vi "CRYTS Step Unflatten.vi"(9 "Sequence Name":string, 10 "Version":u16, 11 "Flattened Steps":string) -> (3 "Unflattened Steps":T2[](array[typedef]) {"Repeat State Array"."Start" format="%#_5g"; "Y dB ref" format="%.1f"; "Y data" items=["dB", "Lin"]; "Start" format="%#_5g"})   [LabVIEW 2013]
uses:
  CRYSystem/Typedef Control/CRYStep.ctl
panel:
  in  "Version2,3":T1(array[cluster])
  in  "Version1":T3(array[cluster])
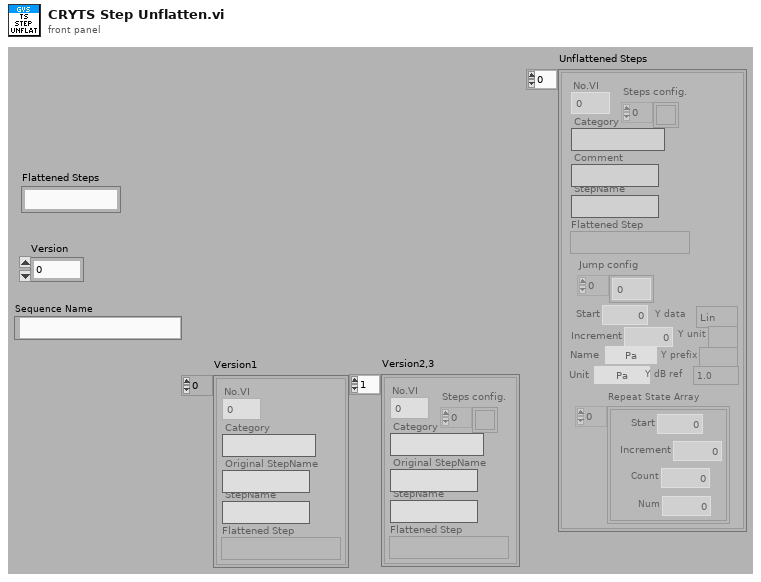
[diagram p1: front panel]
types:
  T1 = cluster{"No.VI":u16, "Category":string, "StepName":string, "Seq setup flattened":string, "Original StepName":string, "Steps config.":bool[]}[]
  T2 = typedef "CRYStep.ctl" = cluster{"No.VI":i32, "Category":string, "StepName":string, "Seq setup flattened":string, "Comment":string, "Steps config.":bool[], "Jump config":i32[], "Start":dbl, "Increment":dbl, "Name":string, "Unit":string, "Y data":u16, "Y prefix":string, "Y dB ref":dbl, "Y unit":string, "Repeat State Array":cluster{"Start":dbl, "Increment":dbl, "Count":i32, "Num":i32}[]}
  T3 = cluster{"No.VI":u16, "Category":string, "StepName":string, "Seq setup flattened":string, "Original StepName":string}[]
  T4 = cluster{"No.VI":i32, "Category":string, "StepName":string, "Seq setup flattened":string, "Original StepName":string, "Steps config.":bool[], "Jump config":i32[], "Start":dbl, "Increment":dbl, "Name":string, "Unit":string, "Y data":u16, "Y prefix":string, "Y dB ref":dbl, "Y unit":string}[]
  T5 = cluster{"Start":dbl, "Increment":dbl, "Count":i32, "Num":i32}[]
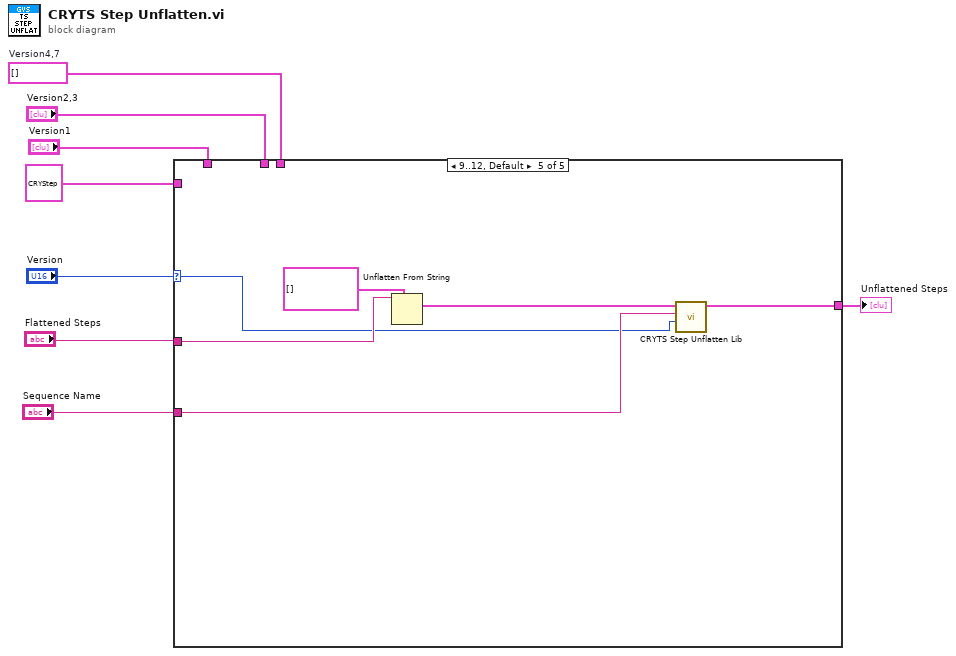
[diagram p0: block diagram]
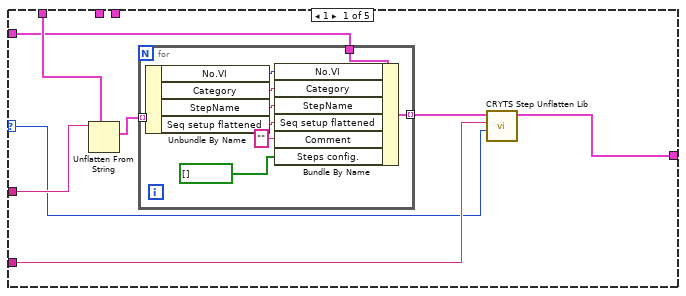
[diagram p2: hidden frame]
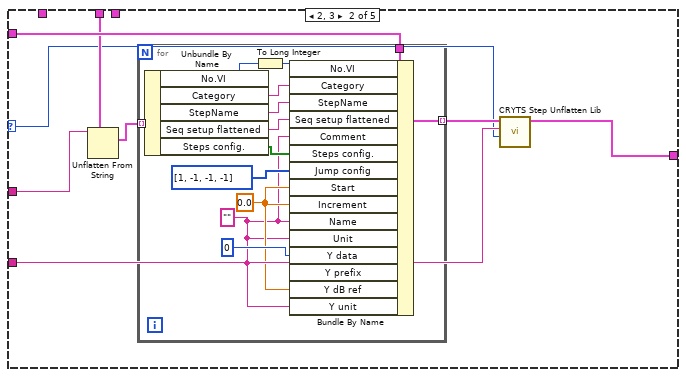
[diagram p3: hidden frame]
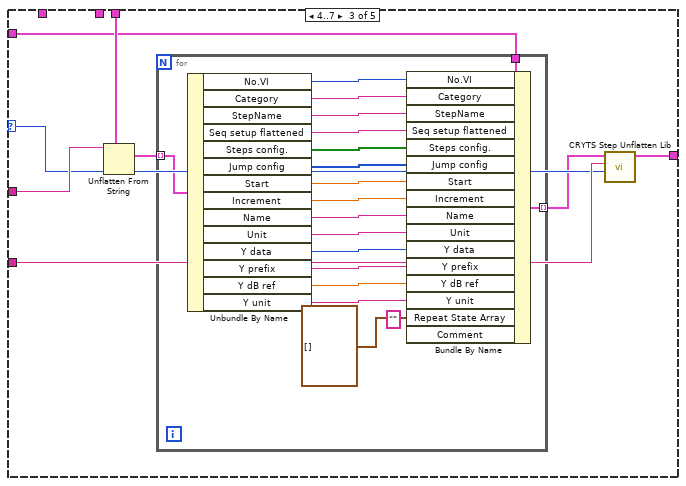
[diagram p4: hidden frame]
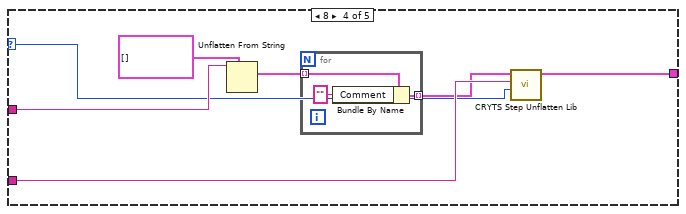
[diagram p5: hidden frame]
diagram:
  w1 = T4 []  # Version4,7
  n1 = case shown="9..12, Default" "Version" {
    selector: "Version" -> [w9 w26 w51 w76 w85]
    tunnel: [w11 w28 w53 w78 w87] -> w4
    tunnel: "Flattened Steps" -> [w16 w32 w54 w79 w88]
    tunnel: "Version1" -> [w14 _ _ _ _]
    tunnel: T2 {"No.VI"=0, "Category"="", "StepName"="", "Seq setup flattened"="", "Comment"="", "Steps config."=[], "Jump config"=[], "Start"=0.0, "Increment"=0.0, "Name"="", "Unit"="", "Y data"=0, "Y prefix"="", "Y dB ref"=0.0, "Y unit"="", "Repeat State Array"=[]} ("Step") -> [w13 w31 w48 _ _]
    tunnel: "Version2,3" -> [_ w30 _ _ _]
    tunnel: "Sequence Name" -> [w10 w27 w52 w77 w86]
    tunnel: w1 -> [_ _ w50 _ _]
    frame 1 {
      n2 = Unflatten From String(type=w14, binary string=w16) -> (value=w15:T3)  [unwired: 1 in, 4 out]
      n3 = for {
        tunnel: w15 -> [w24] mode=indexing
        tunnel: w13 -> [w25]
        tunnel: [w18] -> w12 mode=indexing
        n4 = Unbundle By Name(w24) -> ("No.VI"=w23:u16, "Category"=w22:string, "StepName"=w21:string, "Seq setup flattened"=w20:string)
        n5 = Bundle By Name(cluster=w25, "No.VI"=w23, "Category"=w22, "StepName"=w21, "Seq setup flattened"=w20, "Comment"="", "Steps config."=bool[] []) -> (w18:T2)
      }
      n6 = call "CRYTS Step Unflatten Lib.vi"("Version"=w9, "Sequence Name"=w10, "Steps In"=w12) -> ("Steps Out"=w11:T2[])  [unwired: 8 in]
    }
    frame 2, 3 {
      n7 = Unflatten From String(type=w30, binary string=w32) -> (value=w33:T1)  [unwired: 1 in, 4 out]
      n8 = for {
        tunnel: w33 -> [w45] mode=indexing
        tunnel: w31 -> [w46]
        tunnel: [w40] -> w29 mode=indexing
        w34 = "" ("Name")
        w36 = 0.0 ("Start")
        n9 = Unbundle By Name(w45) -> ("No.VI"=w44:u16, "Category"=w43:string, "StepName"=w42:string, "Seq setup flattened"=w41:string, "Steps config."=w39:bool[])
        n10 = To Long Integer(number=w44) -> (32bit integer=w35:i32)
        n11 = Bundle By Name(cluster=w46, "No.VI"=w35, "Category"=w43, "StepName"=w42, "Seq setup flattened"=w41, "Comment"=w34, "Steps config."=w39, "Jump config"=i32[] [1, -1, -1, -1], "Start"=w36, "Increment"=w36, "Name"=w34, "Unit"=w34, "Y data"=u16 0, "Y prefix"=w34, "Y dB ref"=w36, "Y unit"=w34) -> (w40:T2)
      }
      n12 = call "CRYTS Step Unflatten Lib.vi"("Version"=w26, "Sequence Name"=w27, "Steps In"=w29) -> ("Steps Out"=w28:T2[])  [unwired: 8 in]
    }
    frame 4..7 {
      n13 = Unflatten From String(type=w50, binary string=w54) -> (value=w49:T4)  [unwired: 1 in, 4 out]
      n14 = for {
        tunnel: w49 -> [w73] mode=indexing
        tunnel: w48 -> [w72]
        tunnel: [w71] -> w47 mode=indexing
        n15 = Unbundle By Name(w73) -> ("No.VI"=w70:i32, "Category"=w69:string, "StepName"=w68:string, "Seq setup flattened"=w67:string, "Steps config."=w66:bool[], "Jump config"=w65:i32[], "Start"=w64:dbl, "Increment"=w63:dbl, "Name"=w62:string, "Unit"=w61:string, "Y data"=w60:u16, "Y prefix"=w59:string, "Y dB ref"=w58:dbl, "Y unit"=w57:string)
        n16 = Bundle By Name(cluster=w72, "No.VI"=w70, "Category"=w69, "StepName"=w68, "Seq setup flattened"=w67, "Steps config."=w66, "Jump config"=w65, "Start"=w64, "Increment"=w63, "Name"=w62, "Unit"=w61, "Y data"=w60, "Y prefix"=w59, "Y dB ref"=w58, "Y unit"=w57, "Repeat State Array"=T5 [], "Comment"="") -> (w71:T2)
      }
      n17 = call "CRYTS Step Unflatten Lib.vi"("Version"=w51, "Sequence Name"=w52, "Steps In"=w47) -> ("Steps Out"=w53:T2[])  [unwired: 8 in]
    }
    frame 8 {
      n18 = Unflatten From String(type=T2[] [], binary string=w79) -> (value=w75:T2[])  [unwired: 1 in, 4 out]
      n19 = for {
        tunnel: w75 -> [w83] mode=indexing
        tunnel: [w81] -> w74 mode=indexing
        n20 = Bundle By Name(cluster=w83, "Comment"="") -> (w81:T2)
      }
      n21 = call "CRYTS Step Unflatten Lib.vi"("Version"=w76, "Sequence Name"=w77, "Steps In"=w74) -> ("Steps Out"=w78:T2[])  [unwired: 8 in]
    }
    frame 9..12, Default {
      n22 = Unflatten From String(type=T2[] [], binary string=w88) -> (value=w84:T2[])  [unwired: 1 in, 4 out]
      n23 = call "CRYTS Step Unflatten Lib.vi"("Version"=w85, "Sequence Name"=w86, "Steps In"=w84) -> ("Steps Out"=w87:T2[])  [unwired: 8 in]
    }
  }
  "Unflattened Steps" <- w4
